vi "TDAC control.vi"(1 "Voltages before":dbl[](array[numeric]), 4 "Ramp?":bool, 5 "Same?":bool, 6 "Step size":dbl, 8 "error in":errorcluster, 9 "Set voltages":dbl[](array[numeric]), 10 "Channels":string[](array[string]), 11 "Handle in":i32) -> (0 "error out":errorcluster, 2 "TDAC voltages":dbl[](array[numeric]), 3 "Handle out":i32)   [LabVIEW 2018]
panel:
  # "This subVI is used to set the voltages of the high voltage\npower supplies by controlling the output from the TDAC channels\nof the LabJack."
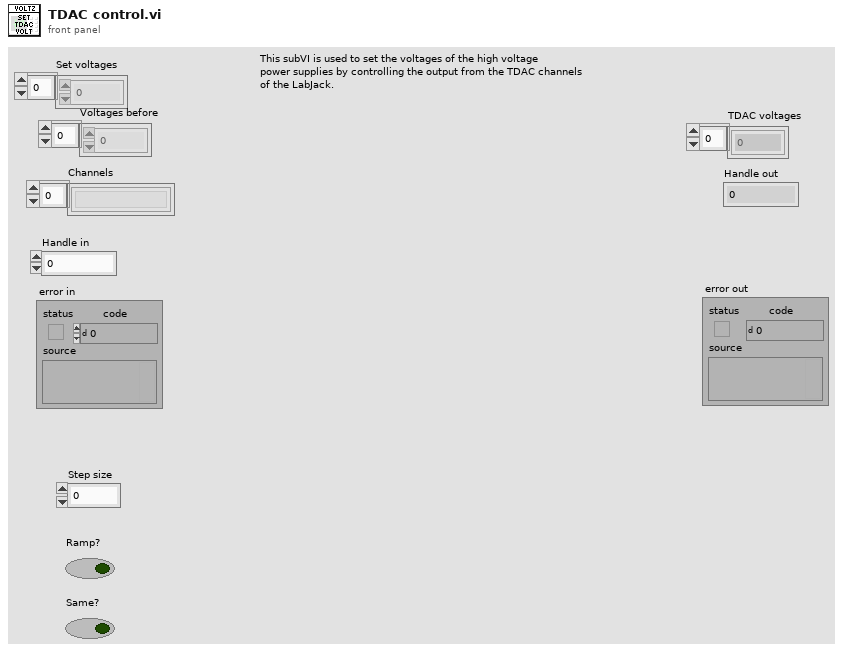
[diagram p1: front panel]
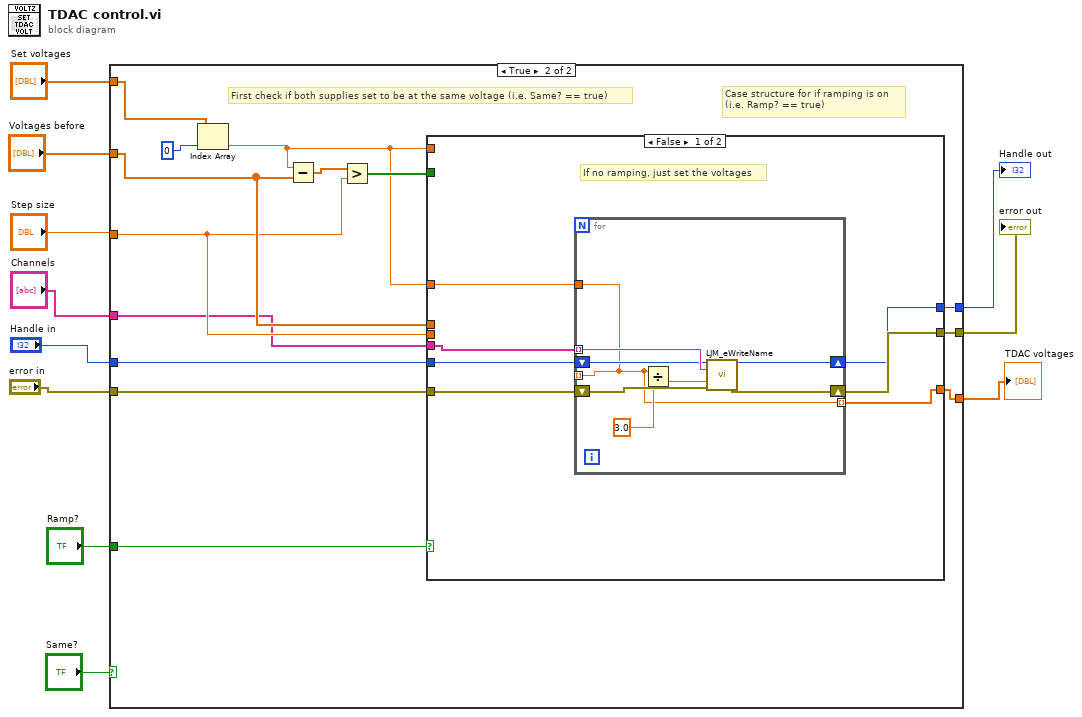
[diagram p0: block diagram]
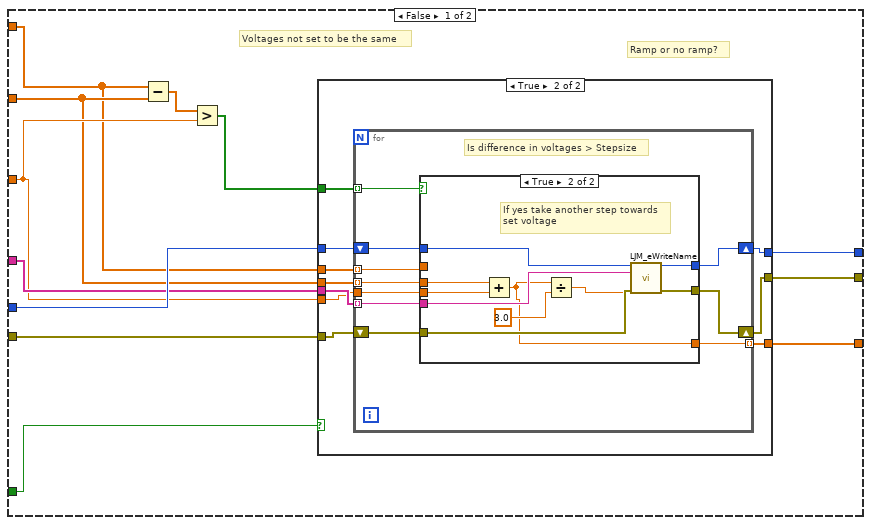
[diagram p2: hidden frame]
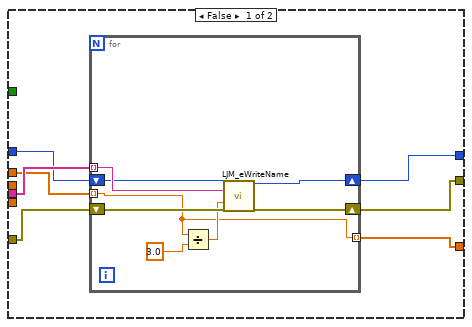
[diagram p3: hidden frame]
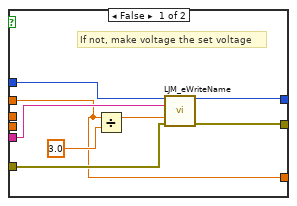
[diagram p4: hidden frame]
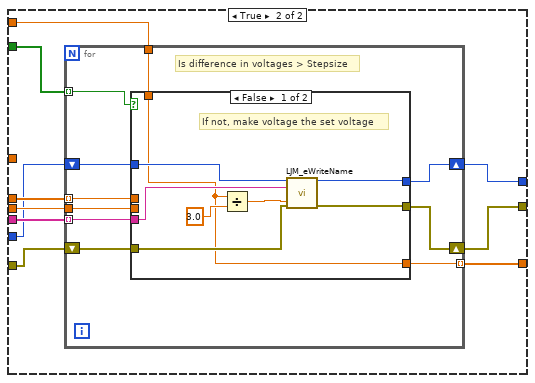
[diagram p5: hidden frame]
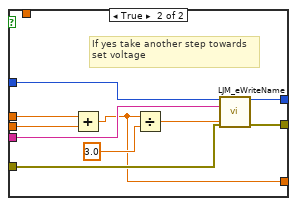
[diagram p6: hidden frame]
diagram:
  n1 = case shown="True" "Same?" {
    tunnel: "Voltages before" -> [w17 w86]
    tunnel: "Set voltages" -> [w16 w79]
    tunnel: "Step size" -> [w18 w85]
    tunnel: "Ramp?" -> [w22 w88]
    tunnel: "error in" -> [w13 w84]
    tunnel: "Channels" -> [w19 w83]
    tunnel: "Handle in" -> [w20 w82]
    tunnel: [w14 w81] -> w3
    tunnel: [w15 w80] -> w2
    tunnel: [w12 w78] -> w1
    frame False {
      # "Ramp or no ramp?"
      # "Voltages not set to be the same"
      n2 = Subtract(x=w16, y=w17) -> (x-y=w23:dbl[])
      n3 = Greater?(x=w23, y=w18) -> (0:w21:bool[])
      n4 = case shown="True" w22 {
        tunnel: w21 -> [_ w48]
        tunnel: w20 -> [w29 w47]
        tunnel: w19 -> [w30 w46]
        tunnel: w18 -> [_ w45]
        tunnel: w17 -> [_ w44]
        tunnel: w16 -> [w28 w43]
        tunnel: [w27 w42] -> w15
        tunnel: [w26 w41] -> w14
        tunnel: w13 -> [w25 w40]
        tunnel: [w24 w39] -> w12
        frame False {
          n5 = for {
            tunnel: w30 -> [w38] mode=indexing
            tunnel: w28 -> [w31] mode=indexing
            shift-right: [w34] -> w26
            shift-left: w29 -> [w37]
            shift-right: [w35] -> w27
            shift-left: w25 -> [w36]
            tunnel: [w31] -> w24 mode=indexing
            n6 = Divide(x=w31, y=3.0) -> (x/y=w32:dbl)
            n7 = call "LJM_eWriteName.vi"("Handle In"=w37, "Name"=w38, "Value"=w32, "error in"=w36) -> ("Handle Out"=w34:i32, "error out"=w35:errorcluster)  [unwired: 10 in]
          }
        }
        frame True {
          n8 = for {
            tunnel: w44 -> [w58] mode=indexing
            tunnel: w45 -> [w57]
            tunnel: w46 -> [w56] mode=indexing
            shift-right: [w54] -> w41
            shift-left: w47 -> [w55]
            shift-right: [w53] -> w42
            shift-left: w40 -> [w52]
            tunnel: w43 -> [w51] mode=indexing
            tunnel: w48 -> [w50] mode=indexing
            tunnel: [w49] -> w39 mode=indexing
            # "Is difference in voltages > Stepsize"
            n9 = case shown="True" w50 {
              tunnel: w58 -> [_ w76]
              tunnel: w57 -> [_ w75]
              tunnel: w52 -> [w64 w73]
              tunnel: w56 -> [w63 w72]
              tunnel: w55 -> [w62 w71]
              tunnel: [w66 w70] -> w54
              tunnel: [w65 w69] -> w53
              tunnel: w51 -> [w59 _]
              tunnel: [w59 w67] -> w49
              frame False {
                # "If not, make voltage the set voltage"
                n10 = Divide(x=w59, y=3.0) -> (x/y=w61:dbl)
                n11 = call "LJM_eWriteName.vi"("Handle In"=w62, "Name"=w63, "Value"=w61, "error in"=w64) -> ("Handle Out"=w66:i32, "error out"=w65:errorcluster)  [unwired: 10 in]
              }
              frame True {
                # "If yes take another step towards\nset voltage"
                n12 = Add(x=w76, y=w75) -> (x+y=w67:dbl)
                n13 = Divide(x=w67, y=3.0) -> (x/y=w68:dbl)
                n14 = call "LJM_eWriteName.vi"("Handle In"=w71, "Name"=w72, "Value"=w68, "error in"=w73) -> ("Handle Out"=w70:i32, "error out"=w69:errorcluster)  [unwired: 10 in]
              }
            }
          }
        }
      }
    }
    frame True {
      # "Case structure for if ramping is on\n(i.e. Ramp? == true)"
      # "First check if both supplies set to be at the same voltage (i.e. Same? == true)"
      n15 = Index Array(array=w79, index=0) -> (element=w77:dbl)
      n16 = Subtract(x=w77, y=w86) -> (x-y=w89:dbl[])
      n17 = Greater?(x=w89, y=w85) -> (0:w87:bool[])
      n18 = case shown="False" w88 {
        tunnel: w87 -> [_ w115]
        tunnel: w86 -> [_ w114]
        tunnel: w85 -> [_ w113]
        tunnel: w84 -> [w95 w108]
        tunnel: w83 -> [w97 w112]
        tunnel: w82 -> [w96 w111]
        tunnel: [w93 w110] -> w81
        tunnel: [w94 w109] -> w80
        tunnel: [w92 w107] -> w78
        tunnel: w77 -> [_ w106]
        tunnel: w77 -> [w91 _]
        frame False {
          # "If no ramping, just set the voltages"
          n19 = for {
            tunnel: w97 -> [w105] mode=indexing
            tunnel: [w98] -> _ mode=indexing
            shift-right: [w101] -> w93
            shift-left: w96 -> [w104]
            shift-right: [w102] -> w94
            shift-left: w95 -> [w103]
            tunnel: [w98] -> w92 mode=indexing
            tunnel: w91 -> [w98]
            n20 = Divide(x=w98, y=3.0) -> (x/y=w100:dbl)
            n21 = call "LJM_eWriteName.vi"("Handle In"=w104, "Name"=w105, "Value"=w100, "error in"=w103) -> ("Handle Out"=w101:i32, "error out"=w102:errorcluster)  [unwired: 10 in]
          }
        }
        frame True {
          n22 = for {
            tunnel: w115 -> [w125] mode=indexing
            tunnel: w114 -> [w124] mode=indexing
            tunnel: w113 -> [w123]
            tunnel: w112 -> [w122] mode=indexing
            shift-right: [w120] -> w110
            shift-left: w111 -> [w121]
            shift-right: [w119] -> w109
            shift-left: w108 -> [w118]
            tunnel: [w117] -> w107 mode=indexing
            tunnel: w106 -> [w116]
            # "Is difference in voltages > Stepsize"
            n23 = case shown="False" w125 {
              tunnel: w124 -> [_ w143]
              tunnel: w123 -> [_ w142]
              tunnel: w118 -> [w131 w140]
              tunnel: w122 -> [w130 w139]
              tunnel: w121 -> [w129 w138]
              tunnel: [w133 w137] -> w120
              tunnel: [w132 w136] -> w119
              tunnel: [w126 w134] -> w117
              tunnel: w116 -> [w126 _]
              frame False {
                # "If not, make voltage the set voltage"
                n24 = Divide(x=w126, y=3.0) -> (x/y=w127:dbl)
                n25 = call "LJM_eWriteName.vi"("Handle In"=w129, "Name"=w130, "Value"=w127, "error in"=w131) -> ("Handle Out"=w133:i32, "error out"=w132:errorcluster)  [unwired: 10 in]
              }
              frame True {
                # "If yes take another step towards\nset voltage"
                n26 = Add(x=w143, y=w142) -> (x+y=w134:dbl)
                n27 = Divide(x=w134, y=3.0) -> (x/y=w135:dbl)
                n28 = call "LJM_eWriteName.vi"("Handle In"=w138, "Name"=w139, "Value"=w135, "error in"=w140) -> ("Handle Out"=w137:i32, "error out"=w136:errorcluster)  [unwired: 10 in]
              }
            }
          }
        }
      }
    }
  }
  "Handle out" <- w3
  "error out" <- w2
  "TDAC voltages" <- w1
